vi "Begin.vi"(8 "error in":errorcluster) -> (0 "error out":errorcluster)   [LabVIEW 2014]
doc: "Called before other user functions, this VI is expected to open initial I/O refnums, load in file data, and do all program initialization. Notice that the <B>error out</B> terminal is simply used for data flow. Wiring it to other structures or subVIs ensures that this VI runs first."
uses:
  <vilib>/Rock Robotics/WPI/DriverStation/WPI_DriverStationRobotMode2.ctl
  <vilib>/Rock Robotics/WPI/Joystick/WPI_JoystickDeviceEnum.ctl
  Robot Global Data.vi
  <vilib>/Rock Robotics/Network Tables/SD Write String Array.vi
  <vilib>/Rock Robotics/WPI/MotorControl/WPI_MotorControlOpenCANTalonSRX.vi
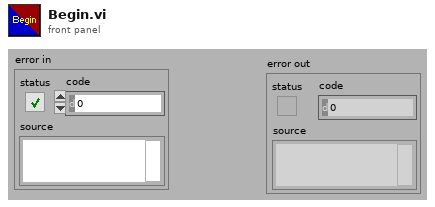
[diagram p1: front panel]
types:
  T1 = typedef "WPI_DriverStationRobotMode2.ctl" = enum16{"Autonomous Disabled", "Autonomous Enabled", "Teleop Disabled", "Teleop Enabled", "Disconnected", "Finish", "Test Disabled", "Test Enabled", "Emergency Stopped"}
  T2 = typedef "WPI_JoystickDeviceEnum.ctl" = enum16{"USB 0", "USB 1", "USB 2", "USB 3", "USB 4", "USB 5"}
  T3 = typedef "WPI_JoystickDevRef.ctl" = cluster{"Device":T2}
  T4 = typedef "WPI_MotorControlDeviceRef.ctl" = cluster{"DeviceStatus":errorcluster, "Type":T5, "PWM":cluster{"Controller":T6, "PWM Channel":T7, "DeadBand":T8}, "CAN":cluster{"Device Number":u8, "Control Mode":T9, "Semaphore":T10, "Max Vout":dbl, "TalonSRX Control Mode":T11}, "Invert":bool, "TransformRef":T12, "InvTransformRef":T12}
  T5 = typedef "WPI_MotorControlType.ctl" = enum16{"PWM", "CAN", "CANTalonSRX"}
  T6 = typedef "FPGA_TypedefDigitalModule.ctl" = enum16{"Controller 1"}
  T7 = typedef "FPGA_DIOPWMChannel.ctl" = enum8{"PWM 0", "PWM 1", "PWM 2", "PWM 3", "PWM 4", "PWM 5", "PWM 6", "PWM 7", "PWM 8", "PWM 9", "PWM MXP 0", "PWM MXP 1", "PWM MXP 2", "PWM MXP 3", "PWM MXP 4", "PWM MXP 5", "PWM MXP 6", "PWM MXP 7", "PWM MXP 8", "PWM MXP 9", "Invalid"}
  T8 = typedef "WPI_PWMDeadband.ctl" = cluster{"Name":string, "maxPositivePwm":i32, "minPositivePwm":i32, "centerPwm":i32, "maxNegativePwm":i32, "minNegativePwm":i32, "angularRange":u16}
  T9 = typedef "WPI_CANJaguar_ControlMode.ctl" = enum8{"Percent VBus", "Current", "Speed", "Position", "Voltage"}
  T10 = typedef "Semaphore RefNum" = refnum<k1>
  T11 = typedef "WPI_CANTalonSRX_APIControlMode.ctl" = enum8{"Percent VBus", "Speed", "Position", "Slave", "Unchanged / Invalid"}
  T12 = typedef "WPI_PWMTransform_ConPane.ctl" = refnum<vi>
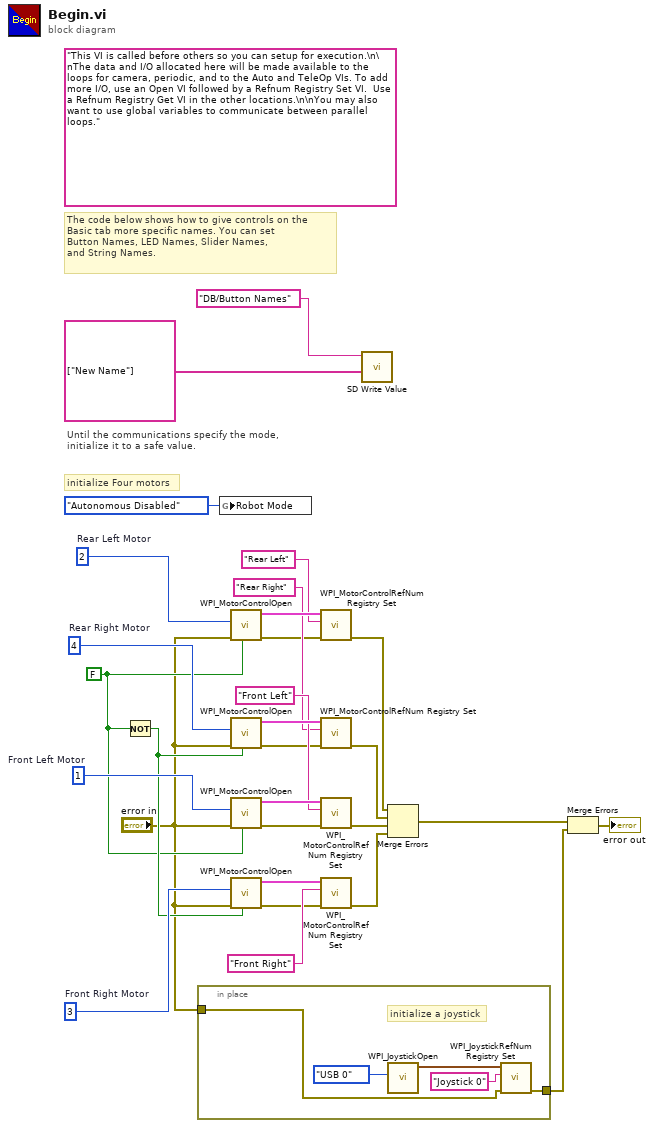
[diagram p0: block diagram]
diagram:
  w11 = FALSE ("Rear Left Motor Inverted")
  w21 = u8 3  # Front Right Motor
  w22 = u8 1  # Front Left Motor
  w23 = u8 4  # Rear Right Motor
  w24 = u8 2  # Rear Left Motor
  (unwired) "This VI is called before others so you can setup for execution.\n\nThe data and I/O allocated here will be made available to the loops for camera, periodic, and to the Auto and TeleOp VIs. To add more I/O, use an Open VI followed by a Refnum Registry Set VI.  Use a Refnum Registry Get VI in the other locations.\n\nYou may also want to use global variables to communicate between parallel loops."
  # "The code below shows how to give controls on the\nBasic tab more specific names. You can set\nButton Names, LED Names, Slider Names,\nand String Names."
  # "Until the communications specify the mode,\ninitialize it to a safe value."
  # "initialize Four motors"
  n1 = Not(x=w11) -> (.not. x?=w12:bool)
  n2 = in-place {
    in-place-border: [w31] -> w26
    in-place-border: "error in" -> [w30]
    # "initialize a joystick"
    n3 = call <vilib>:"WPI_JoystickOpen.vi"("JoystickDevice"=WPI_JoystickDeviceEnum."USB 0") -> ("JoystickDevRef"=w33:T3)  [unwired: 10 in]
    n4 = call <vilib>:"WPI_JoystickRefNum Registry Set.vi"("error in (no error)"=w30, "refnum name"="Joystick 0", "JoystickDevRef"=w33) -> ("error out"=w31:errorcluster)  [unwired: 7 in, 1 out]
  }
  n5 = global write "Robot Global Data.vi" "Robot Mode"(WPI_DriverStationRobotMode2."Autonomous Disabled" ("Robot Mode")) -> ()
  n6 = call-poly <vilib>:"WPI_MotorControlOpen.vi"("Invert"=w11, "error in (no error)"="error in", "Device Number"=w24) -> ("error out"=w10:errorcluster, "MotorControlDeviceRef"=w17:T4)  [unwired: 7 in]
  n7 = call-poly <vilib>:"WPI_MotorControlOpen.vi"("Invert"=w12, "error in (no error)"="error in", "Device Number"=w23) -> ("error out"=w9:errorcluster, "MotorControlDeviceRef"=w18:T4)  [unwired: 7 in]
  n8 = call-poly <vilib>:"WPI_MotorControlOpen.vi"("Invert"=w11, "error in (no error)"="error in", "Device Number"=w22) -> ("error out"=w8:errorcluster, "MotorControlDeviceRef"=w19:T4)  [unwired: 7 in]
  n9 = call-poly <vilib>:"WPI_MotorControlOpen.vi"("Invert"=w12, "error in (no error)"="error in", "Device Number"=w21) -> ("error out"=w7:errorcluster, "MotorControlDeviceRef"=w20:T4)  [unwired: 7 in]
  n10 = call <vilib>:"WPI_MotorControlRefNum Registry Set.vi"("error in (no error)"=w10, "refnum name"="Rear Left", "MotorControlDevRef"=w17) -> ("error out"=w6:errorcluster)  [unwired: 7 in, 1 out]
  n11 = call <vilib>:"WPI_MotorControlRefNum Registry Set.vi"("error in (no error)"=w9, "refnum name"="Rear Right", "MotorControlDevRef"=w18) -> ("error out"=w5:errorcluster)  [unwired: 7 in, 1 out]
  n12 = call <vilib>:"WPI_MotorControlRefNum Registry Set.vi"("error in (no error)"=w8, "refnum name"="Front Left", "MotorControlDevRef"=w19) -> ("error out"=w4:errorcluster)  [unwired: 7 in, 1 out]
  n13 = call <vilib>:"WPI_MotorControlRefNum Registry Set.vi"("error in (no error)"=w7, "refnum name"="Front Right", "MotorControlDevRef"=w20) -> ("error out"=w3:errorcluster)  [unwired: 7 in, 1 out]
  n14 = call-poly <vilib>:"SD Write Value.vi"("String Array"=string[] ["New Name"], "Name"="DB/Button Names") -> ()  [unwired: 8 in, 2 out]
  n15 = Merge Errors(w6, w5, w4, w3) -> (w2:errorcluster)
  n16 = Merge Errors(w2, w26) -> (→"error out":errorcluster)
